vi "MoveItems.vi"(8 "error in (no error)":errorcluster, 11 "CommandLine":string[](array[string])) -> (0 "error out":errorcluster, 2 "test details":string)   [LabVIEW 2019]
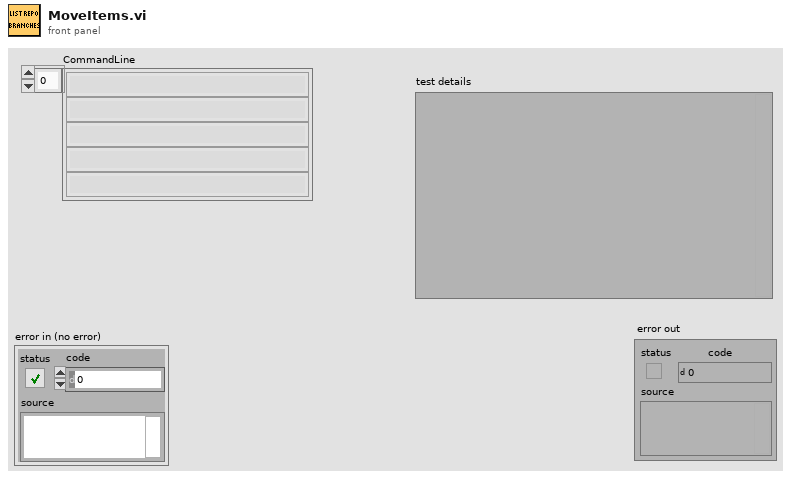
[diagram p1: front panel]
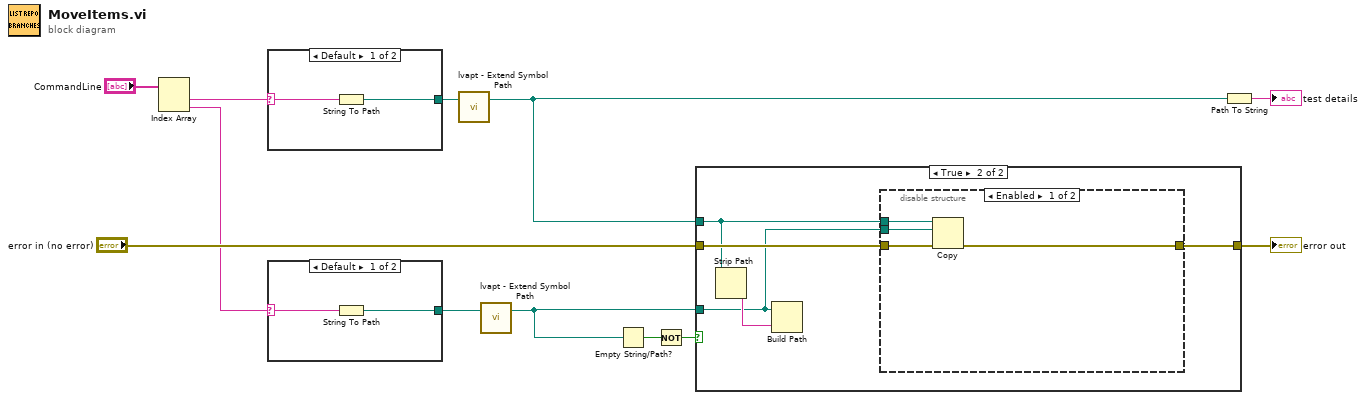
[diagram p0: block diagram]
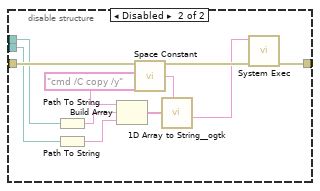
[diagram p3: hidden frame]
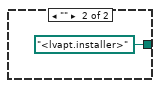
[diagram p4: hidden frame]
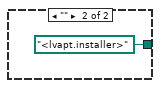
[diagram p5: hidden frame]
diagram:
  n1 = Index Array(array="CommandLine") -> (element #1=w10:string, element #2=w2:string)  [unwired: 2 in]
  n2 = case shown="Default" w10 {
    selector: w10 -> [w14 _]
    tunnel: [w13 path "<lvapt.installer>"] -> w12
    frame Default {
      n3 = String To Path(string=w14) -> (path=w13:path)
    }
    frame "" {
    }
  }
  n4 = case shown="Default" w2 {
    selector: w2 -> [w17 _]
    tunnel: [w16 path "<lvapt.installer>"] -> w8
    frame Default {
      n5 = String To Path(string=w17) -> (path=w16:path)
    }
    frame "" {
    }
  }
  n6 = call <userlib>:"lvapt - Extend Symbol Path.vi"("Symbol Path"=w12) -> ("Resolved Path"=w4:path)  [unwired: 2 in]
  n7 = call <userlib>:"lvapt - Extend Symbol Path.vi"("Symbol Path"=w8) -> ("Resolved Path"=w6:path)  [unwired: 2 in]
  n8 = Empty String/Path?(string/path=w6) -> (empty?=w5:bool)
  n9 = Not(x=w5) -> (.not. x?=w1:bool)
  n10 = case shown="True" w1 {
    tunnel: "error in (no error)" -> [w19 w24]
    tunnel: [w19 w23] -> w7
    tunnel: w4 -> [_ w22]
    tunnel: w6 -> [_ w20]
    frame False {
    }
    frame True {
      n11 = Strip Path(path=w22) -> (name=w21:string)  [unwired: 1 out]
      n12 = Build Path(base path=w20, name or relative path=w21) -> ()  [unwired: 1 out]
      n13 = disable-structure shown="Enabled" {
        disable-tunnel: w24 -> [w28 w37]
        disable-tunnel: [w27 w38] -> w23
        disable-tunnel: w20 -> [w26 w35]
        disable-tunnel: w22 -> [w25 w36]
        frame Enabled {
          n14 = Copy(8:w28, 10:w26, 11:w25) -> (0:w27:errorcluster)  [unwired: 2 in, 2 out]
        }
        frame Disabled {
          n15 = Path To String(path=w36) -> (string=w33:string)
          n16 = Path To String(path=w35) -> (string=w32:string)
          n17 = Build Array("cmd /C copy /y" ("name"), w33, w32) -> (w31:string[])
          n18 = call <vilib>:"Space Constant.vi"() -> ("String"=w30:string)
          n19 = call <userlib>:"1D Array to String__ogtk.vi"("delimiter (Tab)"=w30, "Array of Strings"=w31) -> ("delimited string"=w29:string)  [unwired: 9 in]
          n20 = call <vilib>:"System Exec.vi"("error in (no error)"=w37, "command line"=w29) -> ("error out"=w38:errorcluster)  [unwired: 6 in, 3 out]
        }
      }
    }
  }
  "error out" <- w7
  n21 = Path To String(path=w4) -> (string=→"test details":string)
